vi "finishElementLine.vi"(8 "error in (no error)":errorcluster, 11 "Topic in":refnum<class "Topic.lvclass">) -> (0 "error out":errorcluster, 2 "reachedEnd?":bool, 3 "Topic out":refnum<class "Topic.lvclass">)   [LabVIEW 2016, in "Topic.lvclass"]
uses:
  Topic.lvclass
  Topic.lvclass/Topic.ctl
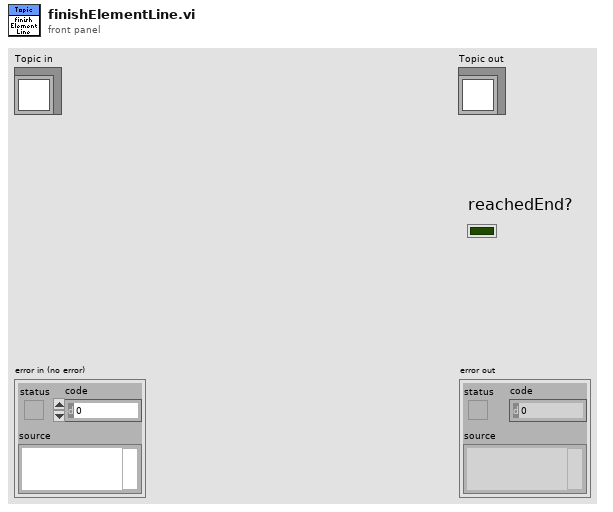
[diagram p1: front panel]
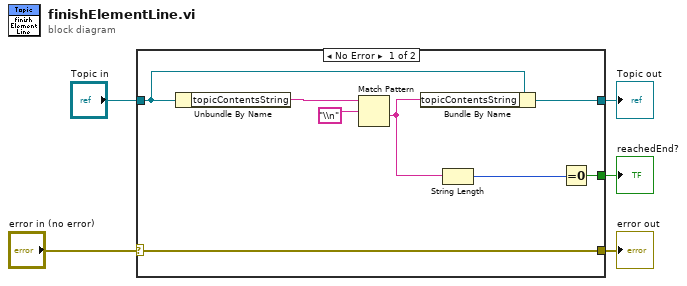
[diagram p0: block diagram]
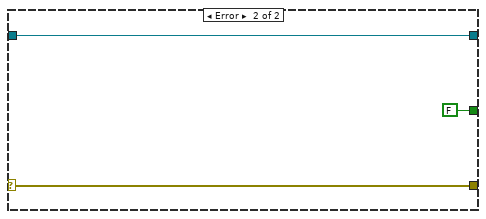
[diagram p2: hidden frame]
diagram:
  n1 = case shown="No Error" "error in (no error)" {
    selector: "error in (no error)" -> [w13 w16]
    tunnel: [w13 w16] -> w4
    tunnel: [w11 w15] -> w2
    tunnel: "Topic in" -> [w12 w15]
    tunnel: [w7 FALSE] -> w1
    frame No Error {
      n2 = Unbundle By Name(w12) -> ("topicContentsString"=w10:string)
      n3 = Match Pattern(string=w10, regular expression="\\n") -> (after substring=w6:string)  [unwired: 1 in, 3 out]
      n4 = Bundle By Name(cluster=w12, "topicContentsString"=w6) -> (w11:refnum<class "Topic.lvclass">)
      n5 = String Length(string=w6) -> (length=w8:i32)
      n6 = Equal To 0?(x=w8) -> (x = 0?=w7:bool)
    }
    frame Error {
    }
  }
  "error out" <- w4
  "Topic out" <- w2
  "reachedEnd?" <- w1
